vi "Timer_Stop.vi"(8 "error in (no error)":errorcluster caption="错误输入（无错误）", 11 "Timer 输入":refnum<class "Timer.lvclass">) -> (0 "error out":errorcluster caption="错误输出", 3 "Timer 输出":refnum<class "Timer.lvclass">)   [LabVIEW 2019, in "Timer.lvclass"]
uses:
  Timer.lvclass
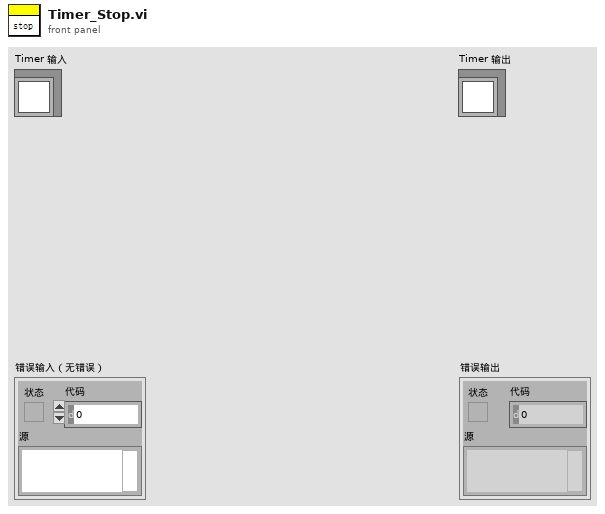
[diagram p1: front panel]
types:
  T1 = typedef "Timer.lvclass/Attribute.ctl" = cluster{"计时？":bool, "计时 (ms)":u32, "停止通知":refnum<notifier>}
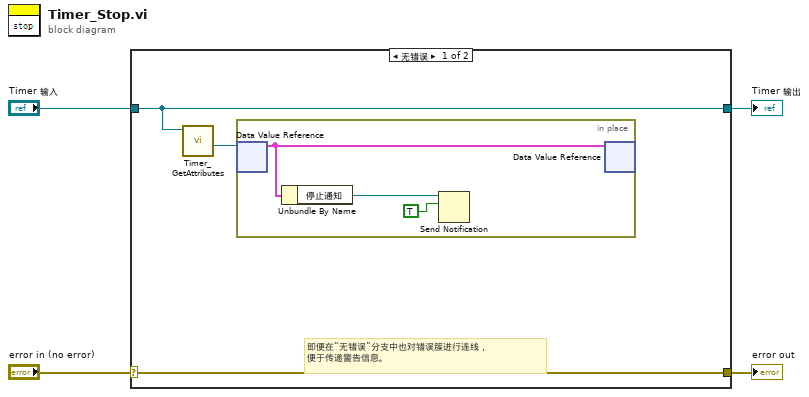
[diagram p0: block diagram]
diagram:
  n1 = case shown="无错误" "error in (no error)" {
    selector: "error in (no error)" -> [w7 w12]
    tunnel: [w7 w12] -> w3
    tunnel: [w6 w11] -> w1
    tunnel: "Timer 输入" -> [w6 w11]
    frame No Error {
      # "即便在“无错误”分支中也对错误簇进行连线，\n便于传递警告信息。"
      n2 = call "Timer_GetAttributes.vi"("Timer 输入"=w6) -> ("数据值引用"=w5:refnum<data-value>)  [unwired: 7 in, 3 out]
      n3 = in-place {
        n4 = in-place-dvr #1(w5) -> (w10:T1)  [unwired: 1 out]
        n5 = Unbundle By Name(w10) -> ("停止通知"=w9:refnum<notifier>)
        n6 = Send Notification(notification=TRUE ("通知"), notifier=w9) -> ()  [unwired: 1 in, 2 out]
        n7 = in-place-dvr #1(w10) -> ()  [unwired: 2 out]
      }
    }
    frame Error {
    }
  }
  "error out" <- w3
  "Timer 输出" <- w1
